vi "Assist Sampling Measure Freq Panel.vi"(8 "error in":errorcluster) -> (0 "error out":errorcluster, 1 "confirmed?":bool, 2 "meas f avg":dbl caption="Measured frequency [Hz]" format="%0_9p")   [LabVIEW 2020]
doc: "This is simple panel for measurement of the frequency by generic counter."
uses:
  drivers/Counter/Counter Type.ctl
  drivers/Counter/Counter Coupling Mode.ctl
  drivers/Counter/Counter Trigger Edge.ctl
  drivers/Counter/Counter Sensitivity.ctl
  varilib/SGUI Assign References Mode.ctl
  drivers/Counter/Counter Freq Mode Setup.ctl
  drivers/Counter/Counter Session.ctl
  varilib/SGUI Assign Multiple Strings With Tags By Label.vi
  drivers/Counter/Counter.lvlib
  varilib/varilib.lvlib
panel:
  in  "External ref 10 MHz":bool
  out "meas f unca":dbl caption="Type A uncertainty [ppm]" format="%#_4f"
  in  "Attenuate":bool
  in  "Filter":bool
  in  "Integration [s]":dbl
  in  "Trigger level [%]":dbl
  in  "Sensitivity":T1=enum."Medium"
  in  "Trigger Slope":T2=enum."Negative"
  in  "Coupling":T3=enum."DC"
  out "idn string":string caption="Identification"
  in  "type":T4 caption="Counter type"
  in  "visa":refnum<visa-resource-name> caption="Counter VISA resource"
  in  "avg":i32=1 caption="Max. averages" min=1
  in  "btn ok":bool
  in  "btn cancel":bool
  in  "btn stop":bool
  in  "btn start":bool
  out "hist f":dbl[](graph) caption="History of the measured frequencies [Hz]"
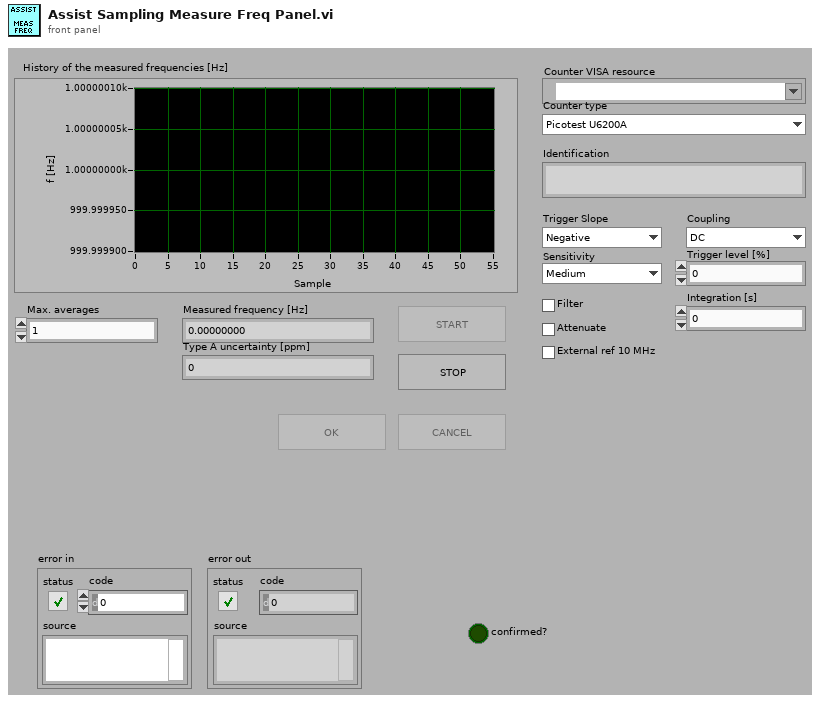
[diagram p1: front panel]
types:
  T1 = typedef "Counter.lvlib/Counter Sensitivity.ctl" = enum16{"High", "Medium", "Low"}
  T2 = typedef "Counter.lvlib/Counter Trigger Edge.ctl" = enum16{"Positive", "Negative"}
  T3 = typedef "Counter.lvlib/Counter Coupling Mode.ctl" = enum16{"AC", "DC"}
  T4 = typedef "Counter.lvlib/Counter Type.ctl" = enum16{"Picotest U6200A", "dummy"}
  T5 = typedef "varilib.lvlib/SGUI Assign References Mode.ctl" = enum16{"Add to stack", "Overwrite", "Release last", "Release ID"}
  T6 = typedef "Counter.lvlib/Counter Session.ctl" = cluster{"VISA":refnum<visa-resource-name>, "type":T4}
  T7 = typedef "Counter.lvlib/Counter Freq Mode Setup.ctl" = cluster{"Coupling (0:AC)":T3, "Trigger Slope (0:Positive)":T2, "Sensitivity (0:High)":T1, "Trigger level [%]":dbl, "Filter":bool, "Attenuate":bool, "Integration [s]":dbl, "Ext clock":bool}
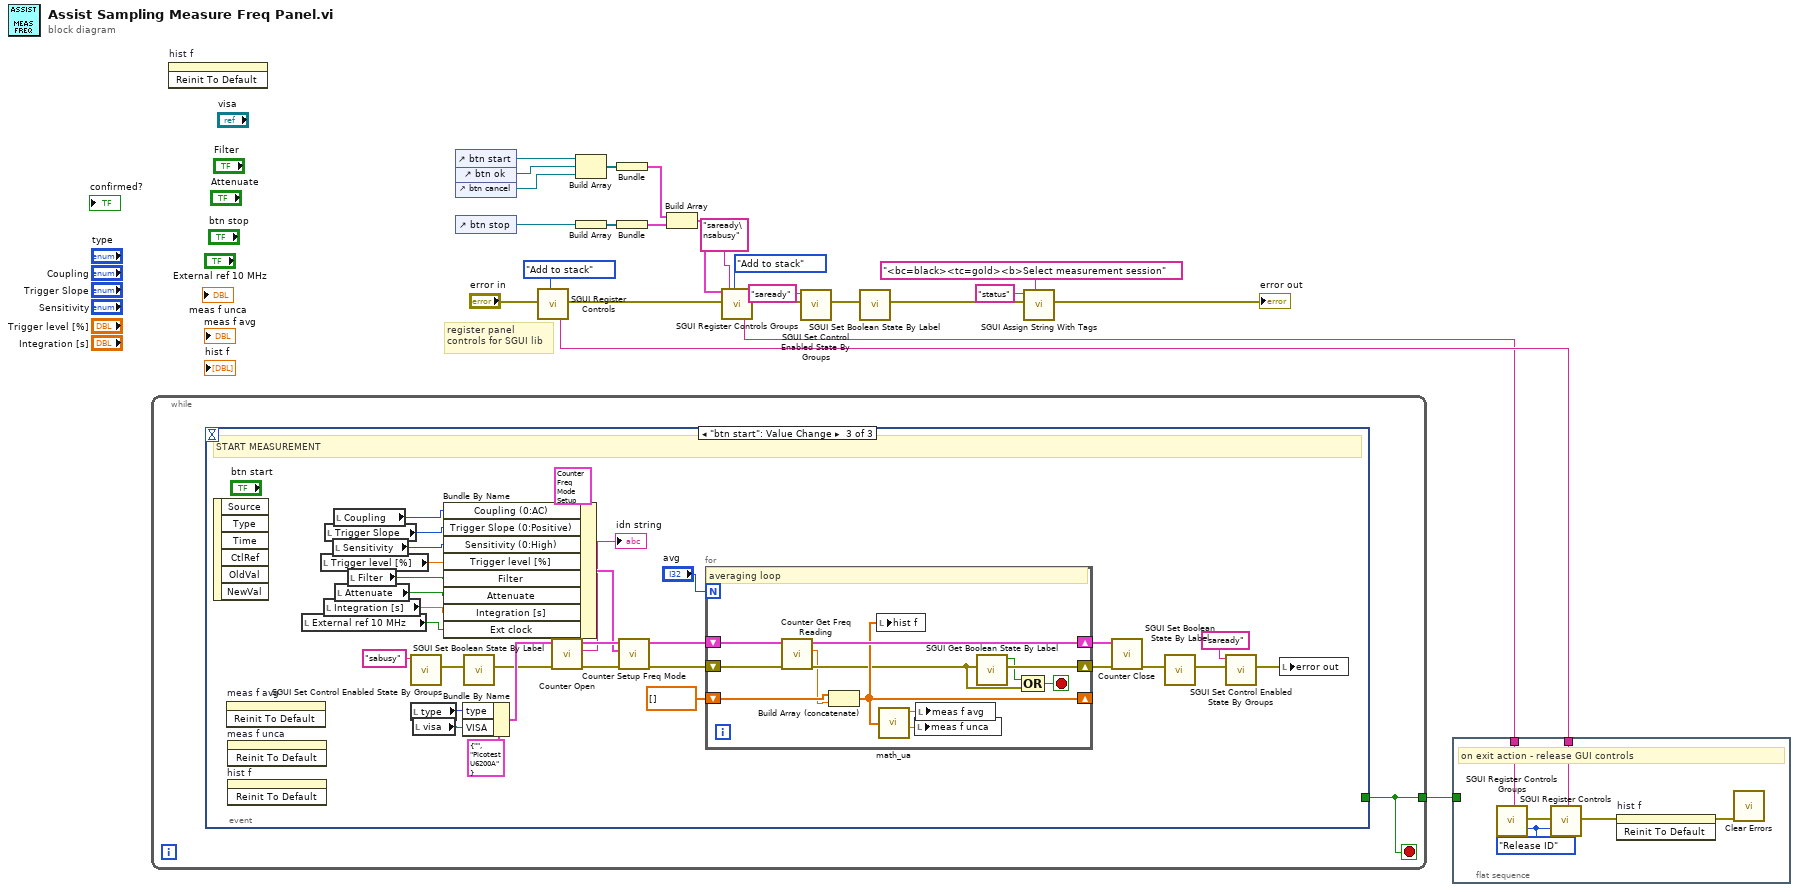
[diagram p0: block diagram]
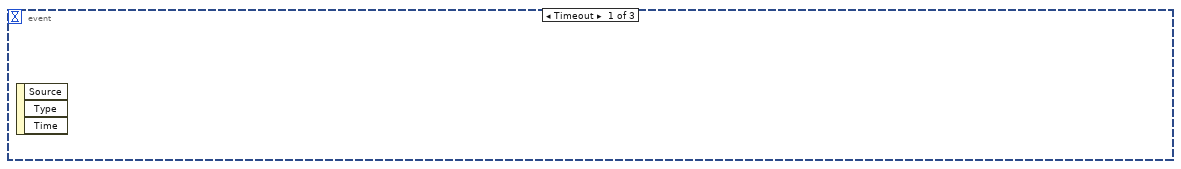
[diagram p2: hidden frame]
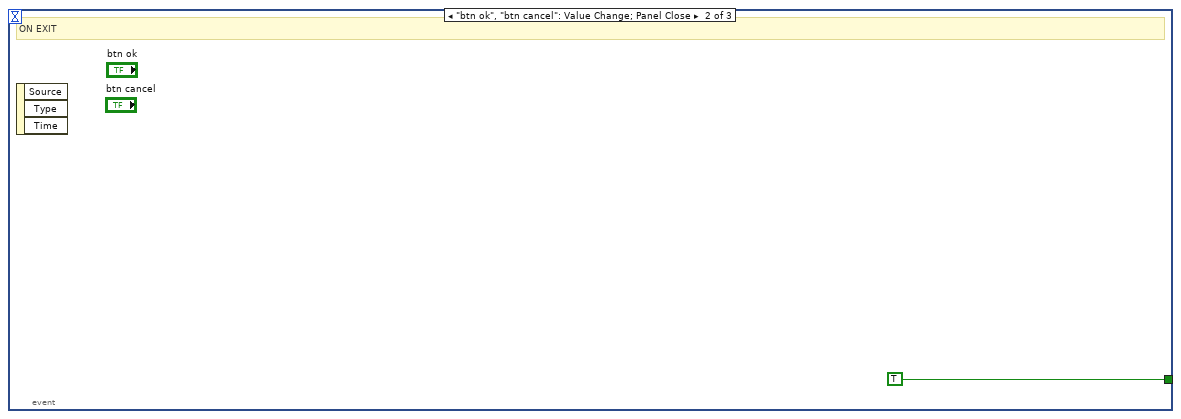
[diagram p3: hidden frame]
diagram:
  # "register panel\ncontrols for SGUI lib"
  n1 = while {
    tunnel: [w25] -> w7
    stop <- w25 stop-if-true
    n2 = event shown="[2] \"btn start\": Value Change" {
      selector: _ -> [_ _ _]
      dyn-events: _ -> [_ _ _]
      timeout: _ -> [_ _ _]
      tunnel: [_ TRUE _] -> w25
      event Timeout {
        n3 = event-data() -> ()  [unwired: 1 in, 3 out]
      }
      event "btn ok", "btn cancel": Value Change; Panel Close {
        # "ON EXIT"
        n4 = event-data() -> ()  [unwired: 1 in, 3 out]
      }
      event "btn start": Value Change {
        # "START MEASUREMENT"
        n5 = event-data() -> ()  [unwired: 1 in, 6 out]
        n6 = invoke on="meas f avg" class="DigNum (strict)" method="Reinit To Default"() -> ()  [unwired: 3 in, 3 out]
        n7 = invoke on="meas f unca" class="DigNum (strict)" method="Reinit To Default"() -> ()  [unwired: 3 in, 3 out]
        n8 = invoke on="hist f" class="WFGraph (strict)" method="Reinit To Default"() -> ()  [unwired: 3 in, 3 out]
        n9 = local read "External ref 10 MHz"() -> (w27:bool)
        n10 = local read "Trigger level [%]"() -> (w38:dbl)
        n11 = local read "Integration [s]"() -> (w35:dbl)
        n12 = local read "Trigger Slope"() -> (w40:T2)
        n13 = local read "Sensitivity"() -> (w39:T1)
        n14 = local read "Coupling"() -> (w41:T3)
        n15 = local read "Attenuate"() -> (w36:bool)
        n16 = local read "Filter"() -> (w37:bool)
        n17 = call "SGUI Set Control Enabled State By Groups.vi"("group name to enable (none)"="sabusy") -> ("error out"=w33:errorcluster)  [unwired: 9 in, 1 out]
        n18 = local read "type"() -> (w46:T4)
        n19 = local read "visa"() -> (w45:refnum<visa-resource-name>)
        n20 = Bundle By Name(cluster=T7 {"Coupling (0:AC)"=enum."DC", "Trigger Slope (0:Positive)"=enum."Negative", "Sensitivity (0:High)"=enum."Medium", "Trigger level [%]"=0.0, "Filter"=FALSE, "Attenuate"=FALSE, "Integration [s]"=0.0, "Ext clock"=FALSE} ("setup"), "Coupling (0:AC)"=w41, "Trigger Slope (0:Positive)"=w40, "Sensitivity (0:High)"=w39, "Trigger level [%]"=w38, "Filter"=w37, "Attenuate"=w36, "Integration [s]"=w35, "Ext clock"=w27) -> (w48:T7)
        n21 = Bundle By Name(cluster=T6 {"VISA"="", "type"=enum."Picotest U6200A"} ("couner session in"), "type"=w46, "VISA"=w45) -> (w44:T6)
        n22 = call "SGUI Set Boolean State By Label.vi"("error in"=w33) -> ("error out"=w32:errorcluster)  [unwired: 9 in, 1 out]
        n23 = call "Counter Open.vi"("error in"=w32, "couner session in"=w44) -> ("error out"=w56:errorcluster, "idn string"=→"idn string":string, "counter session out"=w52:T6)  [unwired: 7 in]
        n24 = call "Counter Setup Freq Mode.vi"("error in"=w56, "setup"=w48, "counter session in"=w52) -> ("error out"=w55:errorcluster, "counter session out"=w51:T6)  [unwired: 7 in]
        n25 = for {
          N: "avg" -> [_]
          shift-right: [w62] -> w54
          shift-left: w55 -> [w68]
          shift-right: [w66] -> w50
          shift-left: w51 -> [w67]
          shift-right: [w64] -> _
          shift-left: dbl[] [] -> [w58]
          stop <- w59 stop-if-true
          # "averaging loop"
          n26 = call "Counter Get Freq Reading.vi"("error in"=w68, "counter session in"=w67) -> ("error out"=w60:errorcluster, "delta t [s]"=w57:dbl, "counter session out"=w66:T6)  [unwired: 7 in]
          n27 = Build Array (concatenate)(w58, w57) -> (w64:dbl[])
          n28 = local write "hist f"(w64) -> ()
          n29 = call "math_ua.vi"("x"=w64) -> ("mean(x)"=w65:dbl, "ua(x) [ppm]"=w63:dbl)  [unwired: 2 out]
          n30 = local write "meas f unca"(w63) -> ()
          n31 = local write "meas f avg"(w65) -> ()
          n32 = call "SGUI Get Boolean State By Label.vi"("error in"=w60) -> ("error out"=w62:errorcluster, "binary state out"=w61:bool)  [unwired: 8 in, 1 out]
          n33 = Compound Arithmetic op=OR(w61, w60) -> (w59:bool)
        }
        n34 = call "Counter Close.vi"("error in"=w54, "couner session in"=w50) -> ("error out"=w31:errorcluster)  [unwired: 8 in, 1 out]
        n35 = call "SGUI Set Boolean State By Label.vi"("error in"=w31) -> ("error out"=w30:errorcluster)  [unwired: 9 in, 1 out]
        n36 = call "SGUI Set Control Enabled State By Groups.vi"("error in"=w30, "group name to enable (none)"="saready") -> ("error out"=w29:errorcluster)  [unwired: 8 in, 1 out]
        n37 = local write "error out"(w29) -> ()
      }
    }
  }
  n38 = invoke on="hist f" class="WFGraph (strict)" method="Reinit To Default"() -> ()  [unwired: 3 in, 3 out]
  n39 = control-ref of="btn start"() -> (w5:refnum<vi>)
  n40 = control-ref of="btn ok"() -> (w4:refnum<vi>)
  n41 = control-ref of="btn cancel"() -> (w3:refnum<vi>)
  n42 = control-ref of="btn stop"() -> (w6:refnum<vi>)
  n43 = call "SGUI Register Controls.vi"("error in"="error in", "register mode (overwrite)"=SGUI_Assign_References_Mode."Add to stack") -> ("assigned ID"=w2:string, "error out"=w21:errorcluster)  [unwired: 15 in, 1 out]
  n44 = Build Array(w5, w4, w3) -> (w18:refnum<vi>[])
  n45 = Build Array(w6) -> (w17:refnum<vi>[])
  n46 = Bundle(w18) -> (w15:cluster{refnum<vi>[]})  [unwired: 1 in]
  n47 = Bundle(w17) -> (w16:cluster{refnum<vi>[]})  [unwired: 1 in]
  n48 = Build Array(w15, w16) -> (w19:cluster{refnum<vi>[]}[])
  n49 = call "SGUI Register Controls Groups.vi"("control groups"=w19, "error in"=w21, "groups names"="saready\nsabusy", "register mode (overwrite)"=SGUI_Assign_References_Mode."Add to stack") -> ("assigned ID"=w1:string, "error out"=w14:errorcluster)  [unwired: 14 in]
  n50 = call "SGUI Set Control Enabled State By Groups.vi"("error in"=w14, "group name to enable (none)"="saready") -> ("error out"=w12:errorcluster)  [unwired: 8 in, 1 out]
  n51 = call "SGUI Set Boolean State By Label.vi"("error in"=w12) -> ("error out"=w11:errorcluster)  [unwired: 9 in, 1 out]
  n52 = call-poly "SGUI Assign String With Tags.vi"("error in"=w11, "label(s) (empty)"="status", "string (empty)"="<bc=black><tc=gold><b>Select measurement session") -> ("error out"=→"error out":errorcluster)  [unwired: 7 in, 1 out]
  n53 = flat-sequence {
    tunnel: w7 -> [_]
    tunnel: w2 -> [w70]
    tunnel: w1 -> [w69]
    frame #0 {
      w73 = SGUI_Assign_References_Mode."Release ID" ("register mode (overwrite)")
      # "on exit action - release GUI controls"
      n54 = call "SGUI Register Controls Groups.vi"("register mode (overwrite)"=w73, "controls ID (empty)"=w69) -> ("error out"=w74:errorcluster)  [unwired: 16 in, 1 out]
      n55 = call "SGUI Register Controls.vi"("error in"=w74, "register mode (overwrite)"=w73, "controls ID (empty)"=w70) -> ("error out"=w71:errorcluster)  [unwired: 14 in, 2 out]
      n56 = invoke on="hist f" class="WFGraph (strict)" method="Reinit To Default"(error in=w71) -> (error out=w72:errorcluster)  [unwired: 2 in, 2 out]
      n57 = call <vilib>:"Clear Errors.vi"("error in (no error)"=w72) -> ()  [unwired: 5 in, 2 out]
    }
  }
